vi "Host_test.vi"() -> ()   [LabVIEW 2016]
uses:
  <vilib>/FPGAPlugInAG/PXIe-7972R/niLvFpga_Open_PXIe-7972R.vi
  <vilib>/rvi/interface/common/dynamic/niFpgaDynamicAddResources.vi
  <vilib>/Utility/error.llb/Error Cluster From Error Code.vi
  <vilib>/rvi/errors/niLvFpgaAdjustHostInterfaceError.vi
  <vilib>/FPGAPlugInAG/Dynamic/niLvFpga_Close_Dynamic.vi
  <vilib>/rvi/interface/nirviOpenFPGA/nirviOpenFPGA.xnode
  FPGA Bitfiles/DMAStreamTest_FPGATarget2_Testbuild_DD4SYgM5wYg.lvbitx
  <vilib>/rvi/interface/nirviReadWriteControl/nirviReadWriteControl.xnode
  <vilib>/rvi/interface/nirviMethod/nirviMethod.xnode
  <vilib>/rvi/interface/nirviCloseFPGA/nirviCloseFPGA.xnode
  NiFpgaLv.dll
  <vilib>/rvi/interface/Simulation/niFpgaSimulationCallBeginRW.vi
  <vilib>/FPGAPlugInAG/Dynamic/niLvFpga_ReadFifo_Dynamic.vi
  <vilib>/rvi/errors/niLvFpgaMergeErrorWithErrorCode.vi
panel:
  out "Count":u64
  out "Waveform Graph":u64[](graph)
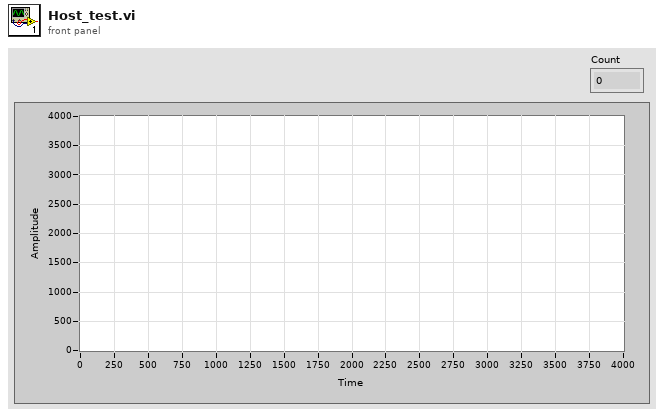
[diagram p1: front panel]
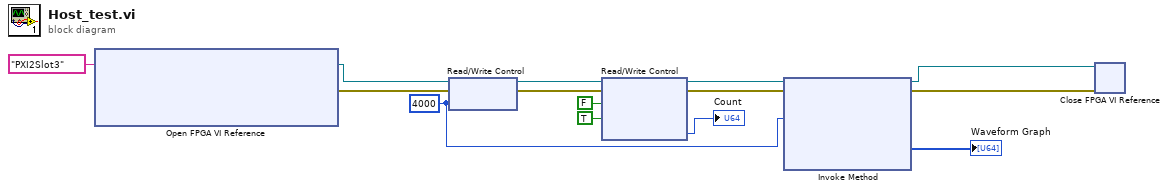
[diagram p0: block diagram]
diagram:
  w3 = u64 4000 ("BatchSize")
  n1 = xnode "Open FPGA VI Reference"("resource name"=tag "PXI2Slot3") -> ("FPGA VI Reference Out"=w11:refnum<k20>, "error out"=w13:errorcluster)  [unwired: 1 in]
  n2 = xnode "Read/Write Control"("FPGA VI Reference In"=w11, "error in"=w13, "BatchSize"=w3) -> ("FPGA VI Reference Out"=w9:refnum<k20>, "error out"=w12:errorcluster)
  n3 = xnode "Read/Write Control"("FPGA VI Reference In"=w9, "error in"=w12, "StartTransfer"=FALSE, "StartTransfer"=TRUE) -> ("FPGA VI Reference Out"=w5:refnum<k20>, "error out"=w10:errorcluster, "Count"=→"Count":u64)
  n4 = xnode "Invoke Method"("FPGA VI Reference In"=w5, "error in"=w10, "Number of Elements"=w3) -> ("FPGA VI Reference Out"=w4:refnum<k20>, "error out"=w6:errorcluster, "Data"=→"Waveform Graph":u64[])  [unwired: 1 in, 1 out]
  n5 = xnode "Close FPGA VI Reference"("FPGA VI Reference In"=w4, "error in"=w6) -> ()  [unwired: 1 out]
